vi "f_5_DiDt.vi"(0 "file path (IN)":path, 1 "Project #":string, 2 "Request #":string, 3 "TEST #":string, 5 "error in (no error)":errorcluster, 6 "ICE":dbl) -> (9 "Dt (us)":dbl, 11 "Di (A)":dbl, 13 "Dt (ns)":dbl, 14 "file path (OUT)":path, 15 "Tr (ns)":dbl, 16 "Di/Dt (A/us)":dbl, 17 "DONE Tr":bool, 18 "DONE Di/Dt ON":bool, 19 "error out":errorcluster)   [LabVIEW 2020]
uses:
  <vilib>/Waveform/WDTOps.llb/WDT Waveform Duration DBL.vi
  Global 1.vi
  <vilib>/Waveform/WDTOps.llb/WDT Get Waveform Subset DBL.vi
  <vilib>/measure/mamon.llb/Trigger Detection for 1 Channel.vi
  <vilib>/Analysis/NI_AALBase.lvlib
  <vilib>/measure/NI_MAPro.lvlib
panel:
  in  "Decision ?":bool
  out "75% Irrm":dbl
  out "50% Ice":dbl
  out "Cursor a : Channel 1":dbl
  out "Cursor b : Channel 1":dbl
  out "Waveform Graph":waveform(dbl)[](graph)
  out "ON Region":waveform(dbl)[](graph) caption="DiDt(A/us)"
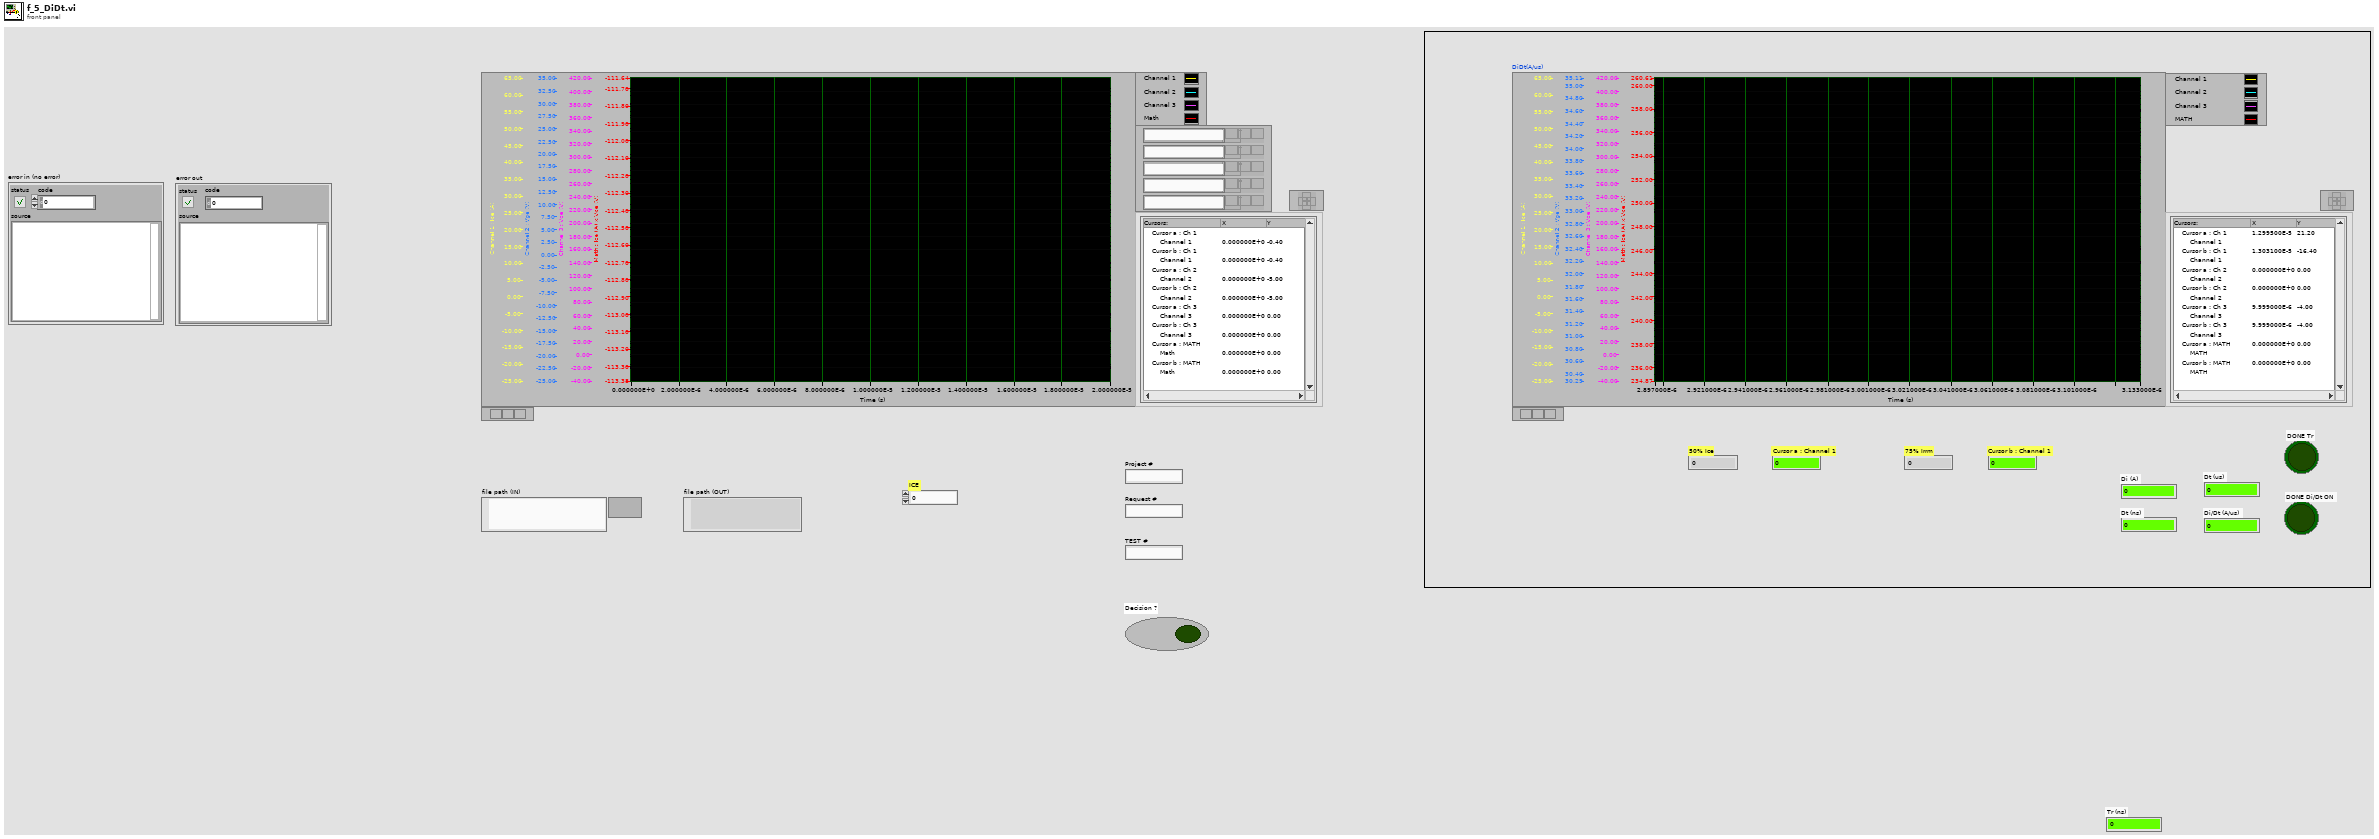
[diagram p1: front panel]
types:
  T1 = enum32{"Invalid", "Standard", "Closed", "Hidden", "Minimized", "Maximized"}
  T2 = typedef "imagedata.ctl" = cluster{"image type":i32, "image depth":i32, "image":u8[], "mask":u8[], "colors":u32[], "Rectangle":cluster{"left":i16, "top":i16, "right":i16, "bottom":i16}}
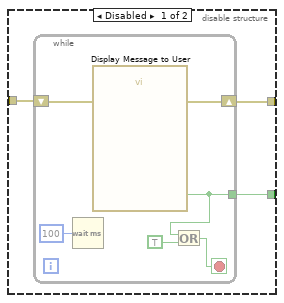
[diagram p2: hidden frame]
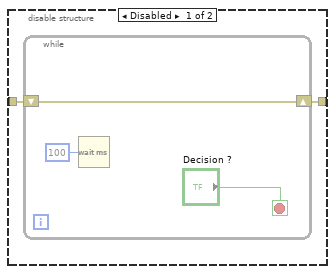
[diagram p7: hidden frame]
diagram:
  w2 = FALSE ("DONE Tdon")
  w1 = 0.0 ("Cursor a : Channel 1")
  w3 = errorcluster {"status"=FALSE, "code"=0, "source"=""} ("error out")
  w4 = waveform(dbl)[] [] ("Waveform Graph")
  n1 = local write "Tr (ns)"(w1) -> ()
  n2 = local write "Cursor a : Channel 1"(w1) -> ()
  n3 = local write "75% Irrm"(w1) -> ()
  n4 = local write "Di (A)"(w1) -> ()
  n5 = local write "Dt (ns)"(w1) -> ()
  n6 = local write "Dt (us)"(w1) -> ()
  n7 = local write "Di/Dt (A/us)"(w1) -> ()
  n8 = local write "Cursor b : Channel 1"(w1) -> ()
  n9 = local write "50% Ice"(w1) -> ()
  n10 = local write "DONE Di/Dt ON"(w2) -> ()
  n11 = local write "Decision ?"(w2) -> ()
  n12 = local write "DONE Tr"(w2) -> ()
  n13 = local write "error out"(w3) -> ()
  n14 = local write "error in (no error)"(w3) -> ()
  n15 = local write "Waveform Graph"(w4) -> ()
  n16 = local write "ON Region"(w4) -> ()
  n17 = flat-sequence {
    tunnel: ["file path (IN)"] -> w10
    tunnel: [w11] -> w9
    tunnel: [w20] -> w8
    tunnel: [w19] -> w7
    tunnel: w10 -> [w22]
    tunnel: w9 -> [w21]
    tunnel: [w261] -> w6
    tunnel: w8 -> [w260]
    tunnel: w7 -> [w259]
    tunnel: [w259] -> w5
    tunnel: w6 -> [w276]
    tunnel: w5 -> [w275]
    frame #0 {
      n18 = control-ref of="This VI"() -> (w16:refnum<vi>)
      n19 = invoke class="VI" method="FP.Open"(reference=w16, error in="error in (no error)", "Activate"=TRUE ("Activate?"), "State"=T1."Maximized") -> (error out=w17:errorcluster)  [unwired: 1 in, 4 out]
      n20 = property class="VI"(reference=w16, error in=w17, "Front Panel.Closeable"=TRUE ("Front Panel Window:Closeable")) -> (error out=w11:errorcluster)  [unwired: 1 out]
    }
    frame #1 {
      n21 = while {
        tunnel: w22 -> [w30]
        shift-right: [w25] -> w20
        shift-left: w21 -> [w29]
        tunnel: [w27] -> w19
        stop <- w24 stop-if-true
        n22 = flat-sequence {
          tunnel: [w64] -> w48
          tunnel: [w65] -> w47
          tunnel: w30 -> [w65]
          tunnel: w29 -> [w64]
          tunnel: w48 -> [w151]
          tunnel: w47 -> [w148]
          tunnel: [w107] -> w46
          tunnel: [w98] -> w45
          tunnel: [w66] -> w23
          tunnel: w46 -> [w188]
          tunnel: [w198] -> w44
          tunnel: w45 -> [w206]
          tunnel: [w206] -> w43
          tunnel: [w194] -> w42
          tunnel: [w197] -> w41
          tunnel: [w183] -> w40
          tunnel: [w189] -> w39
          tunnel: w23 -> [w180]
          tunnel: w44 -> [w218]
          tunnel: [w217] -> w38
          tunnel: w43 -> [w223]
          tunnel: [w223] -> w37
          tunnel: w42 -> [w222]
          tunnel: [w222] -> w36
          tunnel: w41 -> [w221]
          tunnel: [w221] -> w35
          tunnel: w40 -> [w219]
          tunnel: [w219] -> w34
          tunnel: w39 -> [w220]
          tunnel: [w220] -> w33
          tunnel: w38 -> [w232]
          tunnel: w37 -> [w245]
          tunnel: [w245] -> w32
          tunnel: w36 -> [w239]
          tunnel: w35 -> [w240]
          tunnel: w34 -> [w238]
          tunnel: w33 -> [w237]
          tunnel: [w232] -> w31
          tunnel: w32 -> [w250]
          tunnel: w31 -> [w252]
          tunnel: [w251] -> w26
          tunnel: [w250] -> w27
          frame #0 {
            w60 = 0.0 ("Cursor a : Channel 1")
            w61 = waveform(dbl)[] [] ("Waveform Graph")
            w63 = FALSE ("DONE Tdon")
            n23 = local write "DONE Di/Dt ON"(w63) -> ()
            n24 = local write "Decision ?"(w63) -> ()
            n25 = local write "DONE Tr"(w63) -> ()
            n26 = local write "Tr (ns)"(w60) -> ()
            n27 = local write "Cursor a : Channel 1"(w60) -> ()
            n28 = local write "75% Irrm"(w60) -> ()
            n29 = local write "Di (A)"(w60) -> ()
            n30 = local write "Dt (ns)"(w60) -> ()
            n31 = local write "Dt (us)"(w60) -> ()
            n32 = local write "Di/Dt (A/us)"(w60) -> ()
            n33 = local write "Cursor b : Channel 1"(w60) -> ()
            n34 = local write "50% Ice"(w60) -> ()
            n35 = Wait (ms)(milliseconds to wait=u32 400) -> ()  [unwired: 1 out]
            n36 = local write "Waveform Graph"(w61) -> ()
            n37 = local write "ON Region"(w61) -> ()
          }
          frame #1 {
            w75 = u16 1 items=["Samples", "Relative Time"] ("start/duration format")
            w82 = u16 1 items=["Samples", "Relative Time"] ("start/duration format")
            w87 = 0.0 ("number")
            w79 = waveform(dbl) {"t0"=timestamp(0 s since 1904-01-01), "dt"=1.0, "Y"=[]} ("element")
            # "Channel 3"
            # "Channel 1"
            # "t0"
            # "dt"
            # "Ch1"
            n38 = call "3_ReadDatatoWaveform.vi"("error in (no error)"=w151, "file path (IN)"=w148) -> ("error out"=w88:errorcluster, "Waveform Graph"=→"Waveform Graph":waveform(dbl)[], "file path (OUT)"=w98:path, "dt"=w92:dbl, "Ch 3 Data"=w149:dbl[], "Ch 1 Data"=w93:dbl[])  [unwired: 3 in, 1 out]
            n39 = property on="Waveform Graph" class="WFGraph (strict)"(error in=w88, "XScale.Offset"=w87) -> (error out=w69:errorcluster)  [unwired: 1 in, 1 out]
            n40 = To Time Stamp(1:w87) -> (0:w91:timestamp)
            n41 = disable-structure shown="Enabled" {
              disable-tunnel: w91 -> [w171 _]
              disable-tunnel: w92 -> [w170 _]
              disable-tunnel: w93 -> [w169 _]
              disable-tunnel: [w168 _] -> w80
              frame Enabled {
                # "Channel 1"
                n42 = Bundle By Name("Y"=w169, "dt"=w170, "t0"=w171) -> (w168:waveform(dbl))  [unwired: 1 in]
              }
              frame Disabled {
              }
            }
            n43 = disable-structure shown="Enabled" {
              disable-tunnel: w91 -> [w175 _]
              disable-tunnel: w92 -> [w174 _]
              disable-tunnel: w149 -> [w173 _]
              disable-tunnel: [w172 _] -> w72
              frame Enabled {
                # "Channel 3"
                n44 = Bundle By Name("Y"=w173, "dt"=w174, "t0"=w175) -> (w172:waveform(dbl))  [unwired: 1 in]
              }
              frame Disabled {
              }
            }
            n45 = call-poly <vilib>:"Waveform Duration.vi"("error in (no error)"=w69, "waveform in"=w72) -> ("error out"=w78:errorcluster, "duration"=w76:dbl, "waveform out"=w77:waveform(dbl))  [unwired: 7 in]
            n46 = call-poly <vilib>:"Waveform Duration.vi"("error in (no error)"=w69, "waveform in"=w80) -> ("error out"=w86:errorcluster, "duration"=w83:dbl, "waveform out"=w85:waveform(dbl))  [unwired: 7 in]
            n47 = Divide(x=w76, y=2.0) -> (x/y=w74:dbl)
            n48 = Divide(x=w83, y=2.0) -> (x/y=w68:dbl)
            n49 = disable-structure shown="Enabled" {
              disable-tunnel: w80 -> [w165 _]
              disable-tunnel: [w156 _] -> w94
              disable-tunnel: [w154 _] -> w66
              disable-tunnel: w69 -> [w157 _]
              disable-tunnel: w92 -> [w164 _]
              disable-tunnel: w68 -> [w153 _]
              frame Enabled {
                w158 = u16 1 items=["Samples", "Relative Time"] ("start/duration format")
                # "old = 1"
                # "Median-filtered Channel 1"
                # "Median"
                n50 = global read "Global 1.vi" "Median Filter Rank"() -> (w152:i32)
                n51 = Unbundle By Name(w165) -> ("Y"=w167:dbl[])
                n52 = call <vilib>:"Median Filter.vi"("right rank"=w152, "left rank"=w152, "X"=w167) -> ("Filtered X"=w166:dbl[])  [unwired: 7 in, 1 out]
                n53 = Bundle By Name("Y"=w166, "dt"=w164) -> (w155:waveform(dbl))  [unwired: 1 in]
                n54 = call-poly <vilib>:"Waveform Duration.vi"("error in (no error)"=w157, "waveform in"=w155) -> ("error out"=w162:errorcluster, "duration"=w160:dbl, "waveform out"=w161:waveform(dbl))  [unwired: 7 in]
                n55 = Divide(x=w160, y=2.0) -> (x/y=w163:dbl)
                n56 = call-poly <vilib>:"Get Waveform Subset.vi"("start/duration format"=w158, "error in (no error)"=w162, "duration"=w163, "start samples/time"=w153, "waveform in"=w161) -> ("error out"=w156:errorcluster, "waveform out"=w154:waveform(dbl))  [unwired: 1 in, 2 out]
              }
              frame Disabled {
              }
            }
            n57 = call-poly <vilib>:"Get Waveform Subset.vi"("start/duration format"=w75, "error in (no error)"=w78, "duration"=w74, "start samples/time"=w68, "waveform in"=w77) -> ("error out"=w70:errorcluster, "waveform out"=w71:waveform(dbl))  [unwired: 1 in, 2 out]
            n58 = call-poly <vilib>:"Get Waveform Subset.vi"("start/duration format"=w82, "error in (no error)"=w86, "duration"=w68, "start samples/time"=w68, "waveform in"=w85) -> ("error out"=w81:errorcluster, "waveform out"=w67:waveform(dbl))  [unwired: 1 in, 2 out]
            n59 = Build Array(w67, w79, w71, w79) -> (→"ON Region":waveform(dbl)[])
            n60 = Merge Errors(w81, w70, w94) -> (w105:errorcluster)
            n61 = property on="ON Region" class="WFGraph (strict)"(error in=w105) -> (error out=w104:errorcluster, "Width"=w103:u32)  [unwired: 1 in, 1 out]
            n62 = property on="ON Region" class="WFGraph (strict)"(error in=w104, "Caption.Justify"=enum16{"Left", "Center", "Right"}."Left" ("Caption.Justification"), "Caption.Width"=w103, "Caption.FontBold"=TRUE ("Caption.Font:Bold"), "Caption.FontColor"=u32 16860 ("Caption.Font:Color"), "Caption.FontSize"=u32 24 ("Caption.Font:Size"), "Caption.Text"="DiDt(A/us)") -> (error out=w90:errorcluster)  [unwired: 1 in, 1 out]
            n63 = property on="ON Region" class="WFGraph (strict)"(error in=w90, "XScale.Offset"=w68) -> (error out=w89:errorcluster)  [unwired: 1 in, 1 out]
            n64 = property on="ON Region" class="WFGraph (strict)"(error in=w89, "Active Cursor"=u32 0, "Cursor.Cursor X"=0.0 ("Cursor.Cursor Position:Cursor X"), "Cursor.Cursor Y"=0.0 ("Cursor.Cursor Position:Cursor Y"), "Cursor.Visible"=FALSE) -> (error out=w130:errorcluster)  [unwired: 1 in, 1 out]
            n65 = property on="ON Region" class="WFGraph (strict)"(error in=w130, "Active Cursor"=u32 1, "Cursor.Cursor X"=0.0 ("Cursor.Cursor Position:Cursor X"), "Cursor.Cursor Y"=0.0 ("Cursor.Cursor Position:Cursor Y"), "Cursor.Visible"=FALSE) -> (error out=w129:errorcluster)  [unwired: 1 in, 1 out]
            n66 = property on="ON Region" class="WFGraph (strict)"(error in=w129, "Active Cursor"=u32 2, "Cursor.Cursor X"=0.0 ("Cursor.Cursor Position:Cursor X"), "Cursor.Cursor Y"=0.0 ("Cursor.Cursor Position:Cursor Y"), "Cursor.Visible"=FALSE) -> (error out=w128:errorcluster)  [unwired: 1 in, 1 out]
            n67 = property on="ON Region" class="WFGraph (strict)"(error in=w128, "Active Cursor"=u32 3, "Cursor.Cursor X"=0.0 ("Cursor.Cursor Position:Cursor X"), "Cursor.Cursor Y"=0.0 ("Cursor.Cursor Position:Cursor Y"), "Cursor.Visible"=FALSE) -> (error out=w111:errorcluster)  [unwired: 1 in, 1 out]
            n68 = property on="ON Region" class="WFGraph (strict)"(error in=w111, "Active Cursor"=u32 4, "Cursor.Cursor X"=0.0 ("Cursor.Cursor Position:Cursor X"), "Cursor.Cursor Y"=0.0 ("Cursor.Cursor Position:Cursor Y"), "Cursor.Visible"=FALSE) -> (error out=w110:errorcluster)  [unwired: 1 in, 1 out]
            n69 = property on="ON Region" class="WFGraph (strict)"(error in=w110, "Active Cursor"=u32 5, "Cursor.Cursor X"=0.0 ("Cursor.Cursor Position:Cursor X"), "Cursor.Cursor Y"=0.0 ("Cursor.Cursor Position:Cursor Y"), "Cursor.Visible"=FALSE) -> (error out=w109:errorcluster)  [unwired: 1 in, 1 out]
            n70 = property on="ON Region" class="WFGraph (strict)"(error in=w109, "Active Cursor"=u32 6, "Cursor.Cursor X"=0.0 ("Cursor.Cursor Position:Cursor X"), "Cursor.Cursor Y"=0.0 ("Cursor.Cursor Position:Cursor Y"), "Cursor.Visible"=FALSE) -> (error out=w108:errorcluster)  [unwired: 1 in, 1 out]
            n71 = property on="ON Region" class="WFGraph (strict)"(error in=w108, "Active Cursor"=u32 7, "Cursor.Cursor X"=0.0 ("Cursor.Cursor Position:Cursor X"), "Cursor.Cursor Y"=0.0 ("Cursor.Cursor Position:Cursor Y"), "Cursor.Visible"=FALSE) -> (error out=w107:errorcluster)  [unwired: 1 in, 1 out]
            n72 = call <vilib>:"Beep.vi"("use system alert? (T)"=FALSE, "duration (msec)"=u32 200, "frequency (Hz)"=u32 2000) -> ()  [unwired: 9 in]
          }
          frame #2 {
            w185 = u16 0 items=["Falling Edge", "Rising Edge"] ("trigger slope")
            w186 = u16 1 items=["Index", "Time"] ("location mode")
            w192 = u16 0 items=["Falling Edge", "Rising Edge"] ("trigger slope")
            w193 = u16 1 items=["Index", "Time"] ("location mode")
            # "Cursor a : Channel 1"
            # "Cursor b : Channel 1"
            # "Cursor b : Channel 1"
            # "Cursor a : Channel 1"
            # "Cursor b : Channel 1"
            # "Cursor a : Channel 1"
            # "Cursor b : Channel 1"
            # "Cursor a : Channel 1"
            # "End Time 1st Cursor"
            # "End Time 2nd Cursor"
            # "1st PARAMETER : 50% Ice"
            # "Channel 1"
            # "2nd PARAMETER : 75% Irrm"
            # "Channel 1"
            n73 = Divide(x=50.0, y=100.0) -> (x/y=w216:dbl)
            n74 = Multiply(x=w216, y="ICE") -> (x*y=w190:dbl)
            "50% Ice" <- w190
            n75 = Add(x=w190, y=0.0) -> (x+y=w182:dbl)
            n76 = call-poly <vilib>:"Basic Level Trigger Detection.vi"("signal in"=w180, "level"=w182, "location mode"=w193, "error in (no error)"=w188, "trigger slope"=w192) -> ("trigger location"=w189:dbl, "error out"=w187:errorcluster)  [unwired: 8 in, 1 out]
            n77 = property on="ON Region" class="WFGraph (strict)"(error in=w187, "Active Cursor"=u32 0, "Cursor.Cursor X"=w189, "Cursor.Visible"=TRUE, "Cursor.Cursor Name Visible"=TRUE) -> (error out=w202:errorcluster)  [unwired: 1 in, 1 out]
            n78 = property on="ON Region" class="WFGraph (strict)"(error in=w202, "Active Cursor"=u32 0) -> (error out=w178:errorcluster, "Cursor.Cursor Y"=w194:dbl)  [unwired: 1 in, 1 out]
            "Cursor a : Channel 1" <- w194
            n79 = call <vilib>:"Waveform Min Max.vi"("error in (no error)"=w178, "waveform in"=w180) -> ("error out"=w177:errorcluster, "Y min"=w179:dbl)  [unwired: 4 in, 4 out]
            n80 = Divide(x=75.0, y=100.0) -> (x/y=w213:dbl)
            n81 = Multiply(x=w213, y=w179) -> (x*y=w176:dbl)
            "75% Irrm" <- w176
            n82 = call-poly <vilib>:"Basic Level Trigger Detection.vi"("signal in"=w180, "level"=w176, "location mode"=w186, "error in (no error)"=w177, "trigger slope"=w185) -> ("trigger location"=w183:dbl, "error out"=w184:errorcluster)  [unwired: 8 in, 1 out]
            n83 = property on="ON Region" class="WFGraph (strict)"(error in=w184, "Active Cursor"=u32 1, "Cursor.Cursor X"=w183, "Cursor.Visible"=TRUE, "Cursor.Cursor Name Visible"=TRUE) -> (error out=w199:errorcluster)  [unwired: 1 in, 1 out]
            n84 = call <vilib>:"Beep.vi"("use system alert? (T)"=FALSE, "duration (msec)"=u32 200, "frequency (Hz)"=u32 2000) -> ()  [unwired: 9 in]
            n85 = property on="ON Region" class="WFGraph (strict)"(error in=w199, "Active Cursor"=u32 1) -> (error out=w198:errorcluster, "Cursor.Cursor Y"=w197:dbl)  [unwired: 1 in, 1 out]
            "Cursor b : Channel 1" <- w197
          }
          frame #3 {
            n86 = disable-structure shown="Enabled" {
              disable-tunnel: w218 -> [w231 _]
              disable-tunnel: [w230 _] -> w217
              disable-tunnel: w220 -> [w225 _]
              disable-tunnel: w219 -> [w224 _]
              frame Enabled {
                # "2nd Cursor"
                # "1st Cursor"
                n87 = Subtract(x=w225, y=1e-07) -> (x-y=w226:dbl)
                n88 = Add(x=w224, y=1e-07) -> (x+y=w227:dbl)
                n89 = property on="ON Region" class="WFGraph (strict)"(error in=w231, "XScale.Minimum"=w226, "XScale.Maximum"=w227) -> (error out=w230:errorcluster)  [unwired: 1 in, 1 out]
              }
              frame Disabled {
              }
            }
          }
          frame #4 {
            # "us"
            # "ns"
            n90 = Subtract(x=w240, y=w239) -> (x-y=w235:dbl)
            n91 = Subtract(x=w238, y=w237) -> (x-y=w236:dbl)
            n92 = Absolute Value(x=w235) -> (abs(x)=w234:dbl)
            "Di (A)" <- w234
            n93 = Absolute Value(x=w236) -> (abs(x)=w233:dbl)
            n94 = Multiply(x=w233, y=1000000000.0) -> (x*y=→"Tr (ns)" →"Dt (ns)":dbl)
            n95 = Multiply(x=w233, y=1000000.0) -> (x*y=w242:dbl)
            "Dt (us)" <- w242
            n96 = call <vilib>:"Beep.vi"("use system alert? (T)"=FALSE, "duration (msec)"=u32 200, "frequency (Hz)"=u32 2000) -> ()  [unwired: 9 in]
            n97 = Divide(x=w234, y=w242) -> (x/y=→"Di/Dt (A/us)":dbl)
          }
          frame #5 {
            n98 = disable-structure shown="Enabled" {
              disable-tunnel: w252 -> [w254 w258]
              disable-tunnel: [w253 w258] -> w251
              frame Disabled {
                n99 = while {
                  shift-right: [w255] -> w253
                  shift-left: w254 -> [w255]
                  stop <- "Decision ?" stop-if-true
                  n100 = Wait (ms)(milliseconds to wait=u32 100) -> ()  [unwired: 1 out]
                }
              }
              frame Enabled {
              }
            }
          }
        }
        n101 = disable-structure shown="Enabled" {
          disable-tunnel: w26 -> [w51 w58]
          disable-tunnel: [w50 w58] -> w25
          disable-tunnel: [w49 TRUE ("NO")] -> w24
          frame Disabled {
            n102 = while {
              tunnel: [w53] -> w49
              shift-right: [w56] -> w50
              shift-left: w51 -> [w57]
              stop <- w55 stop-if-true
              n103 = Wait (ms)(milliseconds to wait=u32 100) -> ()  [unwired: 1 out]
              n104 = call "Display Message to User"("error in (no error)"=w57) -> ("error out"=w56:errorcluster, "NO"=w53:bool)  [unwired: 9 in]
              n105 = Or(x=w53, y=TRUE) -> (x .or. y?=w55:bool)
            }
          }
          frame Enabled {
          }
        }
        n106 = Wait (ms)(milliseconds to wait=u32 100) -> ()  [unwired: 1 out]
      }
    }
    frame #2 {
      w264 = "_"
      n107 = invoke on="ON Region" class="WFGraph (strict)" method="Get Image"(error in=w260) -> (error out=w268:errorcluster, "image data"=w271:T2)  [unwired: 5 in, 4 out]
      n108 = Concatenate Strings("C:\\TRR_Project\\TRR_Image\\" ("string"), "Project #", w264, "Request #", w264, "TEST #", w264, "DiDton" ("string"), ".png" ("string")) -> (w272:string)
      n109 = String To Path(string=w272) -> (path=w270:path)
      n110 = call <vilib>:"Write PNG File.vi"("error in (no error)"=w268, "image data"=w271, "path to PNG file"=w270) -> ("error out"=w261:errorcluster)  [unwired: 7 in, 1 out]
      "DONE Tr" <- TRUE ("DONE Tdon")
      "DONE Di/Dt ON" <- TRUE ("DONE Di/Dt ON")
    }
    frame #3 {
      n111 = disable-structure shown="Enabled" {
        disable-tunnel: w276 -> [w277 _]
        frame Enabled {
          n112 = control-ref of="This VI"() -> (w278:refnum<vi>)
          n113 = invoke class="VI" method="FP.Close"(reference=w278, error in=w277) -> ()  [unwired: 1 in, 3 out]
        }
        frame Disabled {
        }
      }
      "error out" <- w276
      "file path (OUT)" <- w275
    }
  }
